vi "test Create New Import Routing Channels.vi"(8 "error in (no error)":errorcluster, 11 "TestCase in":refnum<class "Routing and Faulting Import Unit Tests.lvclass">) -> (0 "error out":errorcluster, 3 "TestCase out":refnum<class "Routing and Faulting Import Unit Tests.lvclass">)   [LabVIEW 2017, in "Routing and Faulting Import Unit Tests.lvclass"]
uses:
  Routing and Faulting Import Unit Tests.lvclass
  Shared/Channel States.ctl
  Shared/Routing State.ctl
  Shared/Connection.ctl
  <vilib>/addons/_JKI Toolkits/VI Tester/TestCase.llb/TestCase.lvclass
  <vilib>/NI/NI VeriStand Custom Device Import and Export Tool/ImportExport.lvlib
  <vilib>/NI Veristand/Custom Device Tools/Custom Device Utility Library/Custom Device Utility Library.lvlib
  Shared/Routing and Faulting Shared.lvlib
  Scripting/Routing and Faulting Scripting.lvlib
  C:/Program Files (x86)/National Instruments/LabVIEW 2017/vi.lib/addons/_JKI Toolkits/VI Tester/TestCase.llb/TestCase.lvclass
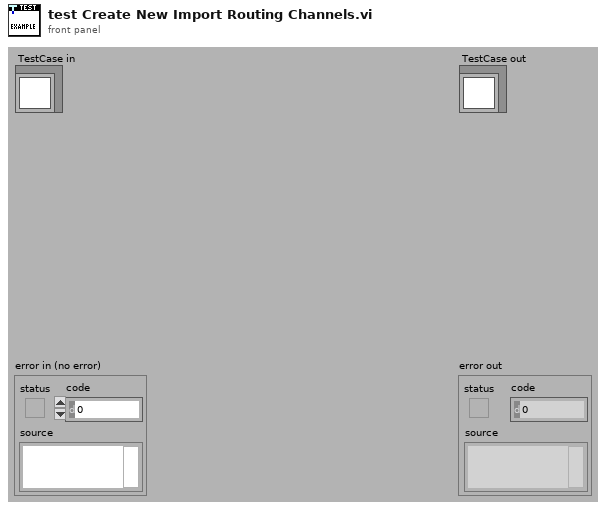
[diagram p1: front panel]
types:
  T1 = typedef "Routing and Faulting Shared.lvlib/Channel States.ctl" = T2[]
  T2 = typedef "Routing and Faulting Shared.lvlib/Routing State.ctl" = cluster{"Name":string, "Description":string, "Value":i32, "Connection List":T3[]}
  T3 = typedef "Routing and Faulting Shared.lvlib/Connection.ctl" = cluster{"Resource":string, "Source":string, "Destination":string}
  T4 = cluster{"Channel Name":string, "Initial State":string, "Description":string, "State Configurations":T1}[]
  T5 = typedef "Custom Device API.lvlib/Custom Device Item Ref.ctl" = u64
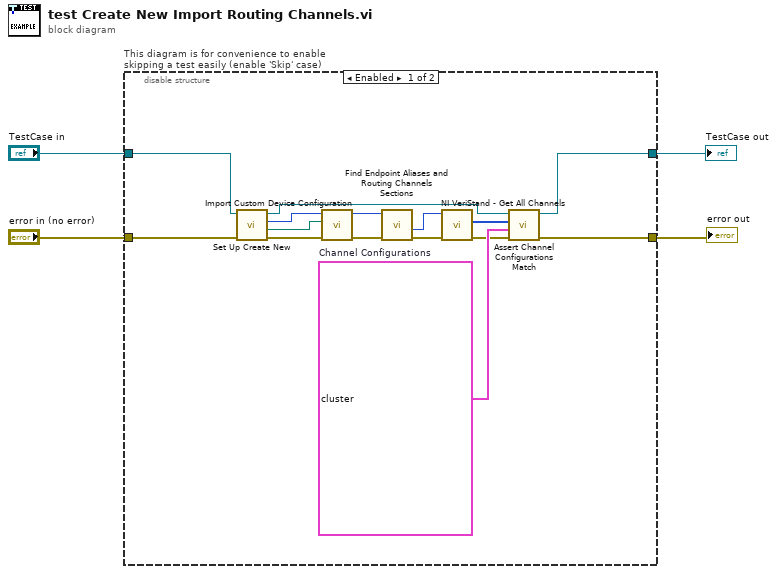
[diagram p0: block diagram]
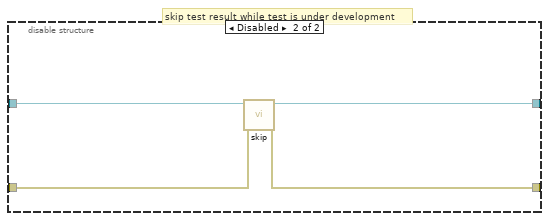
[diagram p2: hidden frame]
diagram:
  n1 = disable-structure "This diagram is for convenience to enable skipping a test easily (enable 'Skip' case)" shown="Enabled" {
    disable-tunnel: "TestCase in" -> [w14 w23]
    disable-tunnel: [w6 w21] -> w1
    disable-tunnel: [w7 w22] -> w3
    disable-tunnel: "error in (no error)" -> [w15 w20]
    frame Enabled {
      w10 = T4 [{"Channel Name"="DefaultValueChan", "Initial State"="", "Description"="", "State Configurations"=[]}, {"Channel Name"="UnchangedChan", "Initial State"="passThrough", "Description"="Should remain the same after import", "State Configurations"=[{"Name"="passThrough", "Description"="passthrough description", "Value"=23, "Connection List"=[{"Resource"="2010A", "Source"="J1Ch0p", "Destination"="J2Ch16p"}]}, {"Name"="addOne", "Description"="addOne description", "Value"=24, "Connection List"=[{"Resource"="2010A", "Source"="J1Ch0p", "Destination"="J2Ch0p"}, {"Resource"="2010B", "Source"="J1Ch0p", "Destination"="J2Ch0p"}]}]}, {"Channel Name"="StateChangeChan", "Initial State"="passThrough", "Description"="Should have a single state called passThrough after import", "State Configurations"=[{"Name"="passThrough", "Description"="passthrough description", "Value"=23, "Connection List"=[{"Resource"="2010A", "Source"="J1Ch0p", "Destination"="J2Ch16p"}]}]}, {"Channel Name"="ImportedChan", "Initial State"="passThrough", "Description"="Should be added to sysdef after import", "State Configurations"=[{"Name"="passThrough", "Description"="passthrough description", "Value"=23, "Connection List"=[{"Resource"="2010A", "Source"="J1Ch0p", "Destination"="J2Ch16p"}]}, {"Name"="addOne", "Description"="addOne description", "Value"=24, "Connection List"=[{"Resource"="2010A", "Source"="J1Ch0p", "Destination"="J2Ch0p"}, {"Resource"="2010B", "Source"="J1Ch0p", "Destination"="J2Ch0p"}]}]}]  # Channel Configurations
      n2 = call "Set Up Create New.vi"("error in (no error)"=w15, "Test Case in"=w14) -> ("error out"=w13:errorcluster, "Import Path"=w11:path, "Routing and Faulting Custom Device Ref"=w12:T5, "Test Case out"=w5:refnum<class "Routing and Faulting Import Unit Tests.lvclass">)  [unwired: 6 in]
      n3 = call <vilib>:"Import Custom Device Configuration.vi"("error in (no error)"=w13, "Path"=w11, "NodeID"=w12) -> ("error out"=w19:errorcluster, "NodeID out"=w18:u64)  [unwired: 6 in, 1 out]
      n4 = call "Find Endpoint Aliases and Routing Channels Sections.vi"("error in (no error)"=w19, "Routing and Faulting Custom Device Ref in"=w18) -> ("error out"=w17:errorcluster, "Routing Channels Ref"=w16:T5)  [unwired: 6 in, 2 out]
      n5 = call <vilib>:"NI VeriStand - Get All Channels.vi"("error in"=w17, "Section Ref in"=w16) -> ("error out"=w8:errorcluster, "Channel Refs"=w9:T5[])  [unwired: 6 in, 2 out]
      n6 = call "Assert Channel Configurations Match.vi"("error in (no error)"=w8, "Channel Configurations"=w10, "Channel Refs"=w9, "Test Case in"=w5) -> ("error out"=w7:errorcluster, "Test Case out"=w6:refnum<class "Routing and Faulting Import Unit Tests.lvclass">)  [unwired: 6 in]
    }
    frame Disabled {
      # "skip test result while test is under development"
      n7 = call <vilib>:"skip.vi"("error in (no error)"=w20, "TestCase in"=w23) -> ("error out"=w22:errorcluster, "TestCase out"=w21:refnum<class "Routing and Faulting Import Unit Tests.lvclass">)  [unwired: 8 in]
    }
  }
  "error out" <- w3
  "TestCase out" <- w1
